vi "solar_voy_def Export (cosmos).vi"(6 "TCPs":T1[](array[typedef]), 8 "error in (no error)":errorcluster, 9 "ALL PACKETS":T3[](array[typedef]) {"last_time" format="%<%H:%M:%S%3u %m/%d/%y>T"}, 10 "Interface Names (\"\" = First Target)":string[](array[string]), 11 "CosmosDir":path) -> (0 "error out":errorcluster, 3 "dup CosmosDir":path)   [LabVIEW 2018]
doc: "This exports all COSMOS packets and tcp interfaces to the corresponding COSMOS configuation folders:\ncosmos\\config\\targets\\TARGET\\cmd_tlm\\TARGET_cmd|tlm.txt - Command & Telemetry definition files\ncosmos\\config\\targets\\TARGET\\cmd_tlm\\cmd_tlm_server.txt - Command & Telemetry server file"
uses:
  solar_voy_def_ctl PATH.ctl
  solar_voy_def_ctl INTERFACE (LINC).ctl
  solar_voy_def_ctl PACKET_ID.ctl
  solar_voy_def_ctl ITEM TYPE.ctl
  type/solar_type Item Type.ctl
  solar_voy_def_ctl ITEM.ctl
  solar_voy_def_ctl PACKET.ctl
  solar_voy_ctl TCP.ctl
  solar_voy_ctl Port Setup.ctl
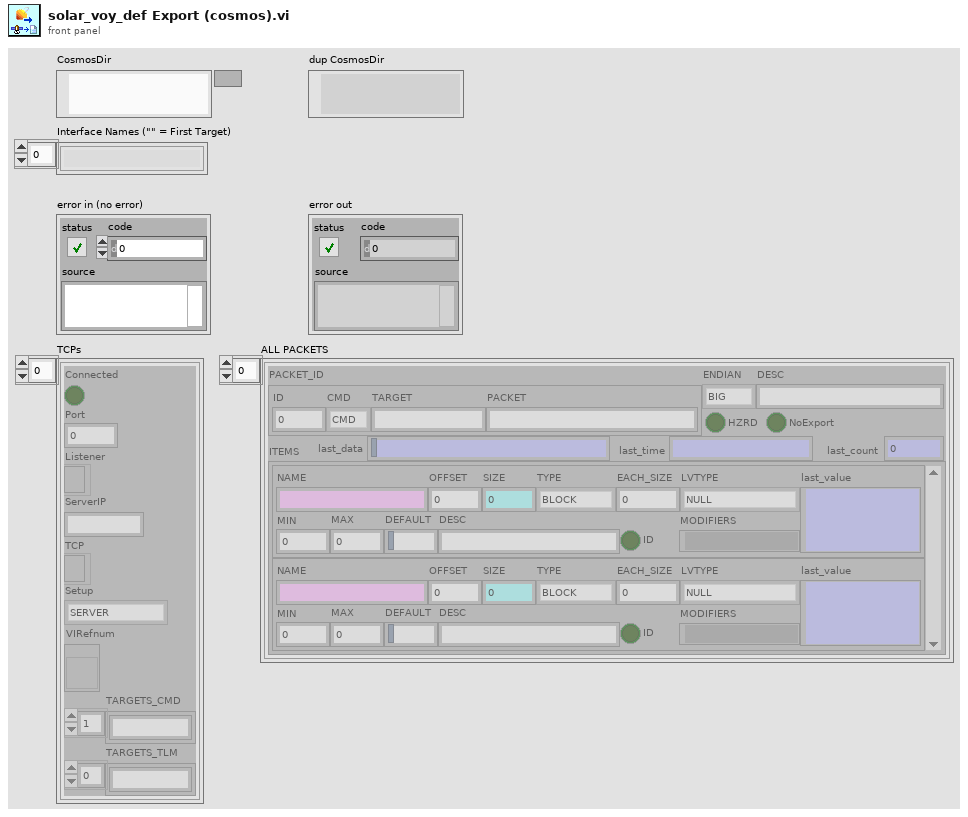
[diagram p1: front panel]
types:
  T1 = typedef "solar_voy_ctl TCP.ctl" = cluster{"Connected":bool, "Port":u16, "Listener":refnum<k5>, "ServerIP":string, "TCP":refnum<k5>, "Setup":T2, "VIRefnum":refnum<vi>, "TARGETS_CMD":string[], "TARGETS_TLM":string[]}
  T2 = typedef "solar_voy_ctl Port Setup.ctl" = enum8{"SERVER", "CLIENT", "SERVER_CMD", "SERVER_TLM"}
  T3 = typedef "solar_voy_def_ctl PACKET.ctl" = cluster{"PACKET_ID":T4, "ENDIAN":enum8{"BIG", "LITTLE"}, "DESC":string, "HZRD":bool, "ITEMS":T5[], "NoExport":bool, "last_time":timestamp, "last_count":u32, "last_data":string}
  T4 = typedef "solar_voy_def_ctl PACKET_ID.ctl" = cluster{"ID":u16, "CMD":enum8{"CMD", "TLM"}, "TARGET":string, "PACKET":string}
  T5 = typedef "solar_voy_def_ctl ITEM.ctl" = cluster{"NAME":string, "OFFSET":i32, "SIZE":i32, "TYPE":T6, "EACH_SIZE":i32, "LVTYPE":T7, "MIN":dbl, "MAX":dbl, "DEFAULT":string, "DESC":string, "ID":bool, "MODIFIERS":variant, "last_value":variant}
  T6 = typedef "solar_voy_def_ctl ITEM TYPE.ctl" = enum8{"BLOCK", "INT", "UINT", "FLOAT", "STRING"}
  T7 = typedef "solar_type Item Type.ctl" = enum16{"NULL", "UNKNOWN", "CLUSTER", "I8", "I16", "I32", "I64", "U8", "U16", "U32", "U64", "U8_ENUM", "U16_ENUM", "U32_ENUM", "SGL", "DBL", "BOOLEAN", "STRING", "PATH", "VISA", "TAG", "TIME", "I8_1D", "I16_1D", "I32_1D", "I64_1D", "U8_1D", "U16_1D", "U32_1D", "U64_1D", "U8_ENUM_1D", "U16_ENUM_1D", "U32_ENUM_1D", "SGL_1D", "DBL_1D", "BOOLEAN_1D", "STRING_1D", "PATH_1D", "VISA_1D", "TAG_1D", "TIME_1D", "I8_2D", "I16_2D", "I32_2D", "I64_2D", "U8_2D", "U16_2D", "U32_2D", "U64_2D", "U8_ENUM_2D", "U16_ENUM_2D", "U32_ENUM_2D", "SGL_2D", "DBL_2D", "BOOLEAN_2D", "STRING_2D", "PATH_2D", "VISA_2D", "TAG_2D", "TIME_2D"}
  T8 = typedef "solar_voy_def_ctl PATH.ctl" = enum8{"..", "config", "config/data", "config/system", "config/targets", "config/targets/TARGET", "config/targets/TARGET/cmd_tlm", "config/targets/TARGET/lib", "config/targets/TARGET/screens", "config/tools", "config/tools/cmd_tlm_server", "config/tools/data_viewer", "config/tools/handbook_creator", "config/tools/launcher", "config/tools/limits_monitor", "config/tools/opengl_builder", "config/tools/script_runner", "config/tools/table_manager", "config/tools/test_runner", "config/tools/tlm_extractor", "config/tools/tlm_grapher", "config/tools/tlm_viewer", "lib", "outputs", "outputs/handbooks", "outputs/logs", "outputs/saved_config", "outputs/tables", "outputs/tmp", "procedures", "tools", "Launcher.bat", "config/system/system.txt", "config/targets/TARGET/cmd_tlm/TARGET_cmd.txt", "config/targets/TARGET/cmd_tlm/TARGET_tlm.txt", "config/targets/TARGET/cmd_tlm_server.txt", "config/targets/TARGET/target.txt", "config/tools/cmd_tlm_server/cmd_tlm_server.txt", "config/tools/data_viewer/data_viewer.txt", "config/tools/handbook_creator/handbook_creator.txt", "config/tools/launcher/launcher.txt", "config/tools/limits_monitor/limits_monitor.txt", "config/tools/opengl_builder/opengl_builder.txt", "config/tools/script_runner/script_runner.txt", "config/tools/table_manager/table_manager.txt", "config/tools/test_runner/test_runner.txt", "config/tools/tlm_extractor/tlm_extractor.txt", "config/tools/tlm_grapher/tlm_grapher.txt", "config/tools/tlm_viewer/tlm_viewer.txt"}
  T9 = typedef "solar_voy_def_ctl INTERFACE (LINC).ctl" = cluster{"name":string, "hostname":string, "port":u16, "handshake_enabled":bool, "response_timeout":dbl, "read_timeout":dbl, "write_timeout":dbl, "length_bitoffset":i32, "length_bitsize":i32, "length_value_offset":i32, "fieldname_guid":string, "endianness":enum8{"BIG", "LITTLE"}, "fieldname_cmd_length":string, "Targets":string[]}
  T10 = typedef "solar_voy_def_ctl INTERFACE.ctl" = cluster{"INTERFACE":string, "TARGETS":string[], "Other":string[]}
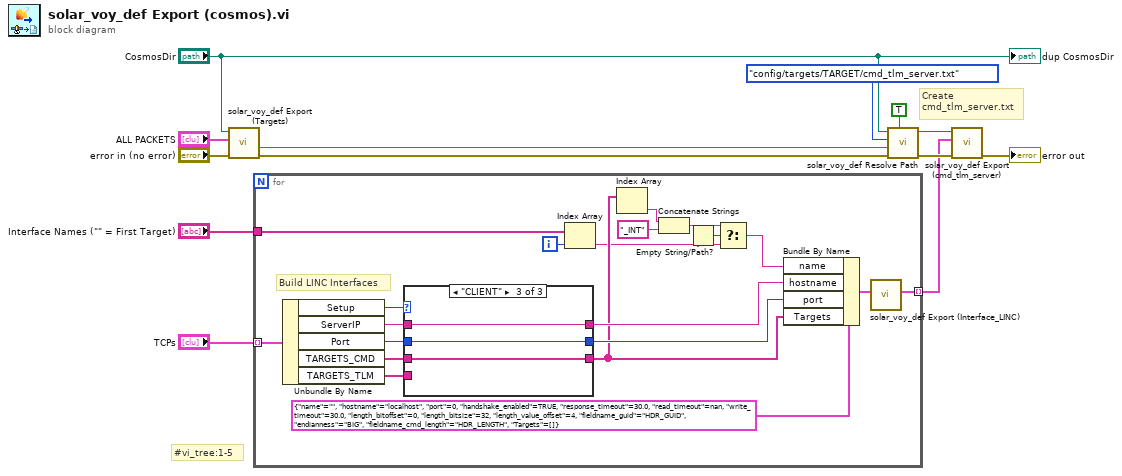
[diagram p0: block diagram]
diagram:
  # "Create \ncmd_tlm_server.txt"
  # "#vi_tree:1-5"
  n1 = call "solar_voy_def Export (Targets).vi"("error in (no error)"="error in (no error)", "ALL PACKETS"="ALL PACKETS", "CosmosDir"="CosmosDir") -> ("error out"=w6:errorcluster, "First Registered Target"=w1:string)  [unwired: 5 in, 2 out]
  n2 = for {
    tunnel: "TCPs" -> [w24] mode=indexing
    tunnel: [w23] -> w3 mode=indexing
    tunnel: "Interface Names (\"\" = First Target)" -> [w16]
    i -> [w14]
    # "Build LINC Interfaces"
    n3 = Unbundle By Name(w24) -> ("Setup"=w31:T2, "ServerIP"=w27:string, "Port"=w29:u16, "TARGETS_CMD"=w26:string[], "TARGETS_TLM"=w25:string[])
    n4 = case shown="\"CLIENT\"" w31 {
      tunnel: [w35 w37 w40] -> w30
      tunnel: w29 -> [w35 w37 w40]
      tunnel: [_ _ w39] -> w28
      tunnel: w27 -> [_ _ w39]
      tunnel: [w34 w36 w38] -> w19
      tunnel: w26 -> [w34 _ w38]
      tunnel: w25 -> [_ w36 _]
      frame "SERVER", "SERVER_CMD" {
        # "\"\" = localhost"
      }
      frame "SERVER_TLM" {
        # "\"\" = localhost"
      }
      frame "CLIENT" {
      }
    }
    n5 = Index Array(array=w16, index=w14) -> (element=w15:string)
    n6 = Index Array(array=w19) -> (element=w18:string)  [unwired: 1 in]
    n7 = Concatenate Strings(w18, "_INT" ("string")) -> (w21:string)
    n8 = Empty String/Path?(string/path=w15) -> (empty?=w20:bool)
    n9 = Select(t=w21, s=w20, f=w15) -> (s? t:f=w17:string)
    n10 = Bundle By Name(cluster=T9 {"name"="", "hostname"="localhost", "port"=0, "handshake_enabled"=TRUE, "response_timeout"=30.0, "read_timeout"=nan, "write_timeout"=30.0, "length_bitoffset"=0, "length_bitsize"=32, "length_value_offset"=4, "fieldname_guid"="HDR_GUID", "endianness"=enum."BIG", "fieldname_cmd_length"="HDR_LENGTH", "Targets"=[]} ("LINC_INTERFACE"), "name"=w17, "hostname"=w28, "port"=w30, "Targets"=w19) -> (w32:T9)
    n11 = call "solar_voy_def Export (Interface_LINC).vi"("LINC_INTERFACE"=w32) -> ("INTERFACE"=w23:T10)  [unwired: 10 in]
  }
  n12 = call "solar_voy_def Resolve Path.vi"("Create Folder? (T)"=TRUE, "error in (no error)"=w6, "TARGET"=w1, "PATH (..=Root)"=solar_voy_def_ctl_PATH."config/targets/TARGET/cmd_tlm_server.txt", "COSMOS_ROOT"="CosmosDir") -> ("error out"=w12:errorcluster, "Resolved Path"=w13:path)  [unwired: 5 in]
  n13 = call "solar_voy_def Export (cmd_tlm_server).vi"("error in (no error)"=w12, "INTERFACES to Merge"=w3, "cmd_tlm_server.txt in"=w13) -> ("error out"=→"error out":errorcluster)  [unwired: 6 in, 2 out]
  "dup CosmosDir" <- "CosmosDir"
